vi "U3 Single AIN Example.vi"() -> (0 "error out":errorcluster)   [LabVIEW 2021]
panel:
  in  "Negative Channel #":i32=199
  in  "quickSample":bool
  in  "longSettling":bool
  in  "Binary":bool
  in  "FirstFound":bool=TRUE
  in  "Address":string="1"
  out "Error Message":string
  out "Value Read":dbl format="%.6f"
  in  "Positive Channel #":i32
  # "Configures and reads 1 analog input."
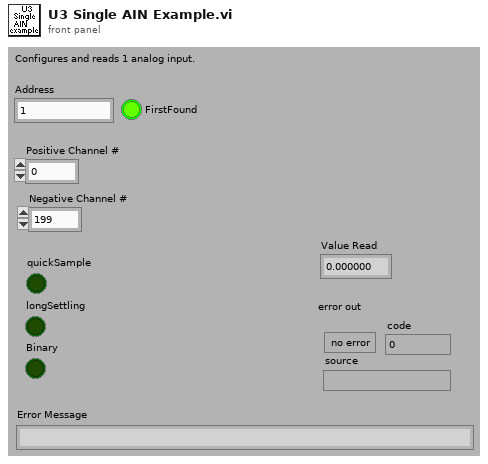
[diagram p1: front panel]
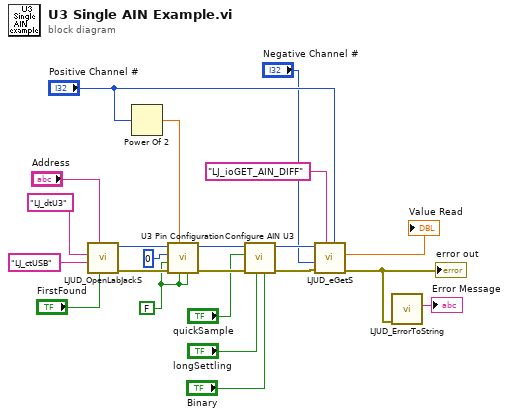
[diagram p0: block diagram]
diagram:
  w5 = FALSE ("Enable DAC1")
  n1 = call "LJUD_OpenLabJackS.vi"("FirstFound"="FirstFound", "Address"="Address", "ConnectionType"="LJ_ctUSB", "DeviceType"="LJ_dtU3") -> ("error out"=w14:errorcluster, "Handle"=w11:i32)  [unwired: 5 in, 1 out]
  n2 = Power Of 2(x="Positive Channel #") -> (2^x=w7:dbl)
  n3 = call "U3 Pin Configuration.vi"("Enable Counter1"=w5, "Enable Counter0"=w5, "FIO/EIO Analog Enable"=w7, "error in"=w14, "Enable DAC1"=w5, "Number of Timers Enabled"=u8 0, "Handle In"=w11) -> ("error out"=w13:errorcluster, "Handle Out"=w10:i32)  [unwired: 3 in]
  n4 = call "Configure AIN U3.vi"("Binary"="Binary", "longSettling"="longSettling", "error in"=w13, "quickSample"="quickSample", "Handle In"=w10) -> ("error out"=w12:errorcluster, "Handle Out"=w9:i32)  [unwired: 5 in]
  n5 = call "LJUD_eGetS.vi"("Channel"="Positive Channel #", "IOType"="LJ_ioGET_AIN_DIFF", "error in"=w12, "x1"="Negative Channel #", "Handle In"=w9) -> ("error out"=w19:errorcluster, "Value Read"=→"Value Read":dbl)  [unwired: 4 in, 1 out]
  "error out" <- w19
  n6 = call "LJUD_ErrorToString.vi"("error in"=w19) -> ("String"=→"Error Message":string)  [unwired: 10 in]
